vi "SMT_Cell Partition.vi"(0 "Traceability 引用句柄":refnum<k24>, 1 "ToCellID":string, 2 "OperatorName":string, 5 "LoadID":string, 7 "FromCellID":string, 9 "FromCircuit":string, 11 "error in (no error)":errorcluster caption="错误输入（无错误）", 12 "ToCircuit":string) -> (4 "Traceability 引用句柄输出":refnum<k24>, 6 "SMT_CellPartition":string, 15 "error out":errorcluster caption="错误输出")   [LabVIEW 2014, in "Traceability.lvlib"]
uses:
  D:/webservice/Traceability.dll
  Traceability.dll
  Traceability.lvlib
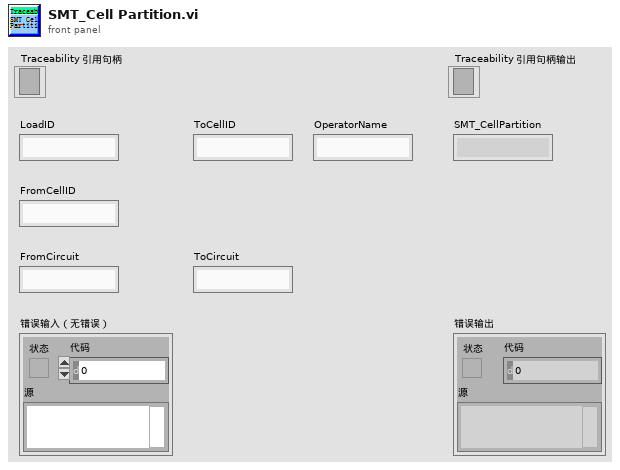
[diagram p1: front panel]
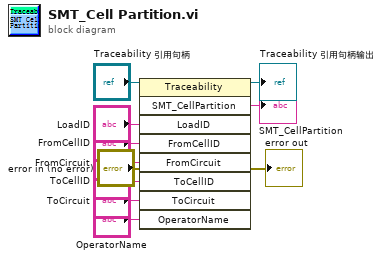
[diagram p0: block diagram]
diagram:
  n1 = invoke class="Traceability" method="SMT_CellPartition"(reference="Traceability 引用句柄", error in="error in (no error)", "LoadID"="LoadID", "FromCellID"="FromCellID", "FromCircuit"="FromCircuit", "ToCellID"="ToCellID", "ToCircuit"="ToCircuit", "OperatorName"="OperatorName") -> (reference out=→"Traceability 引用句柄输出":refnum<k24>, error out=→"error out":errorcluster, "SMT_CellPartition"=→"SMT_CellPartition":string)  [unwired: 1 in, 6 out]
